vi "Recurse.vi"(6 "Error":errorcluster, 7 "Actor":refnum<class "Actor.lvclass">, 11 "Message":refnum<class "Msg.lvclass">) -> (3 "Message":refnum<class "Msg.lvclass">, 4 "Error":errorcluster, 5 "Actor":refnum<class "Actor.lvclass">)   [LabVIEW 2020, in "_Template.lvlib" / "{{Actor}}.lvlib" / "Actor.lvclass"]
uses:
  Actor.lvclass
  Actor.lvclass/Actor.ctl
  jettl/jettl/jettl.lvlib
  jettl/jettl/Msg/Msg.lvclass
panel:
  # "This front panel should not be manipulated."
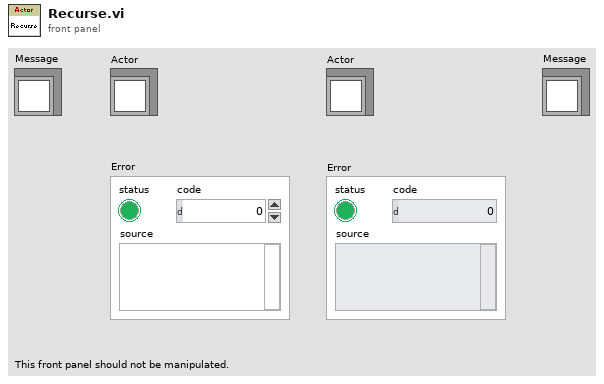
[diagram p1: front panel]
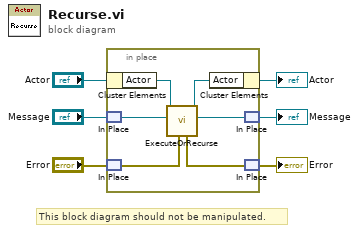
[diagram p0: block diagram]
diagram:
  # "This block diagram should not be manipulated."
  n1 = in-place {
    n2 = in-place-cluster #1("Actor") -> ("Actor"=w12:refnum<class "Actor.lvclass">)
    n3 = in-place-match #2("Message") -> (w8:refnum<class "Msg.lvclass">)
    n4 = in-place-match #3("Error") -> (w10:errorcluster)
    n5 = call "ExecuteOrRecurse.vi"("Error"=w10, "Message"=w8, "Actor"=w12) -> ("Message"=w7:refnum<class "Msg.lvclass">, "Actor"=w11:refnum<class "Actor.lvclass">, "Error"=w9:errorcluster)  [unwired: 6 in]
    n6 = in-place-cluster #1("Actor"=w11) -> (→"Actor":refnum<class "Actor.lvclass">)
    n7 = in-place-match #2(w7) -> (→"Message":refnum<class "Msg.lvclass">)
    n8 = in-place-match #3(w9) -> (→"Error":errorcluster)
  }
